vi "Query OPC.vi"(8 "error in (no error)":errorcluster, 11 "VISA resource name":refnum<visa-resource-name>) -> (0 "error out":errorcluster, 2 "OPC":i32, 3 "VISA resource name out":refnum<visa-resource-name>)   [LabVIEW 2020, in "Rohde&Schwarz CMP LR WPAN Measurement.lvlib"]
doc: "This VI sends OPC query to the instrument. This effectively causes your program to wait in this VI until the instrument has processed all the commands you have sent to it until this point. Use the VI to force the synchronization of the instrument with you program.\n\nAttribute:\n-\n\nRemote-control command:\n*OPC?"
uses:
  <instrlib>/Rohde&Schwarz CMP LR WPAN Measurement/Rohde&Schwarz CMP LR WPAN Measurement.lvlib
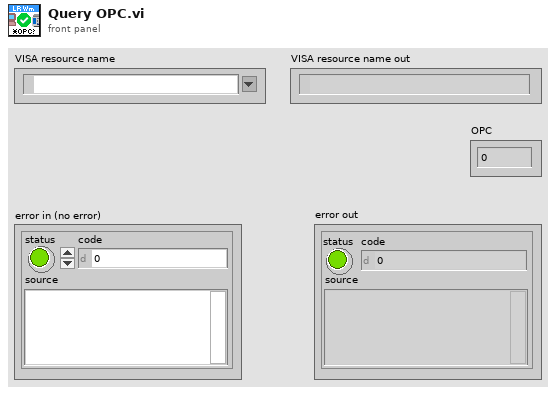
[diagram p1: front panel]
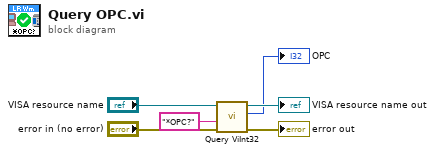
[diagram p0: block diagram]
diagram:
  n1 = call <instrlib>:"Query ViInt32.vi"("error in (no error)"="error in (no error)", "Query"="*OPC?" ("Revision Query Command"), "VISA resource name"="VISA resource name") -> ("error out"=→"error out":errorcluster, "Response Value"=→"OPC":i32, "VISA resource name out"=→"VISA resource name out":refnum<visa-resource-name>)  [unwired: 6 in]
